vi "Model Check.vi"(8 "error in (no error)":errorcluster, 11 "VISA resource name":refnum<visa-resource-name>) -> (0 "error out":errorcluster, 1 "Model":i32(ring) items=["MSO 2000 Series", "DSO 2000 Series", "MSO 3000 Series", "DSO 3000 Series", "MSO 3000T Series", "DSO 3000T Series", "MSO 4000 Series", "DSO 4000 Series", "MSO 6000 Series", "DSO 6000 Series", "1000 Series"], 2 "Not 2000 or 3000 Series":bool, 3 "VISA resource name out":refnum<visa-resource-name>)   [LabVIEW 2023, in "Keysight-DSQx3014T.lvlib"]
doc: "Checks whether the instrument is Agilent InfiniiVision 4000 X-Series Oscilloscopes or not."
uses:
  Keysight-DSQx3014T.lvlib
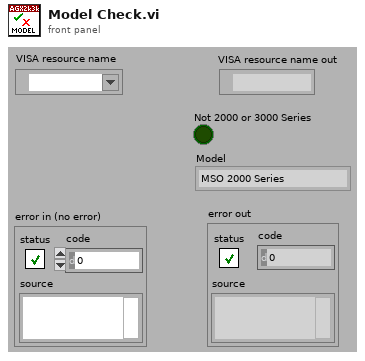
[diagram p1: front panel]
types:
  T1 = typedef "Keysight-DSQx3014T.lvlib/Extended User Data.ctl" = cluster{"X-Series Mode":u16, "Acquisition Type (0: Normal)":i32}
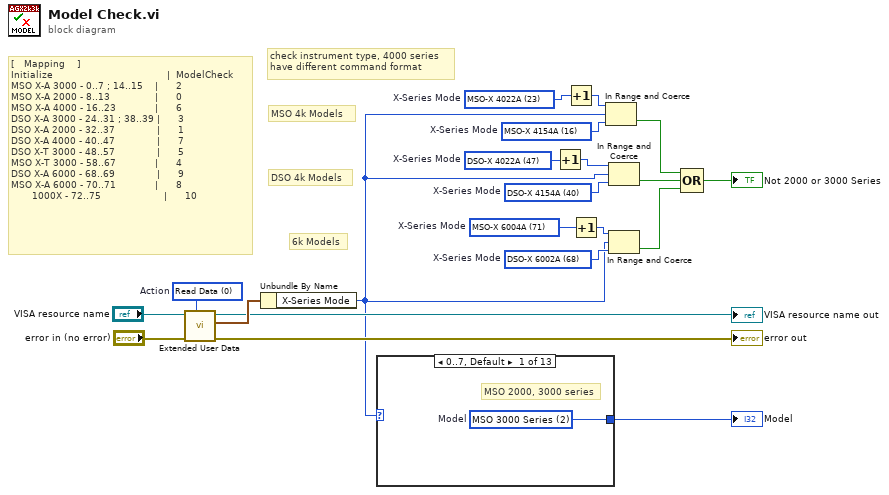
[diagram p0: block diagram]
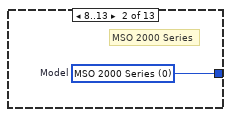
[diagram p2: hidden frame]
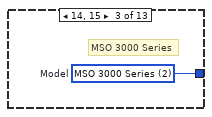
[diagram p3: hidden frame]
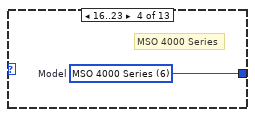
[diagram p4: hidden frame]
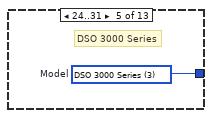
[diagram p5: hidden frame]
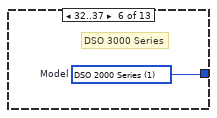
[diagram p6: hidden frame]
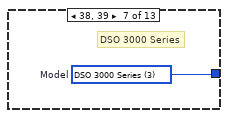
[diagram p7: hidden frame]
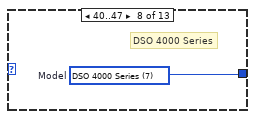
[diagram p8: hidden frame]
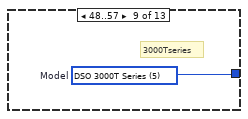
[diagram p9: hidden frame]
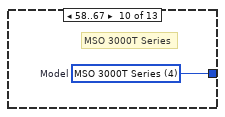
[diagram p10: hidden frame]
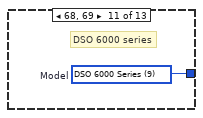
[diagram p11: hidden frame]
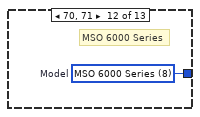
[diagram p12: hidden frame]
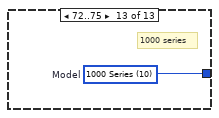
[diagram p13: hidden frame]
diagram:
  w9 = u16 68 items=["MSO-X 3014A", "MSO-X 3024A", "MSO-X 3034A", "MSO-X 3054A", "MSO-X 3012A", "MSO-X 3022A", "MSO-X 3032A", "MSO-X 3052A", "MSO-X 2004A", "MSO-X 2014A", "MSO-X 2024A", "MSO-X 2002A", "MSO-X 2012A", "MSO-X 2022A", "MSO-X 3104A", "MSO-X 3102A", "MSO-X 4154A", "MSO-X 4104A", "MSO-X 4054A", "MSO-X 4034A", "MSO-X 4024A", "MSO-X 4052A", "MSO-X 4032A", "MSO-X 4022A", "DSO-X 3014A", "DSO-X 3024A", "DSO-X 3034A", "DSO-X 3054A", "DSO-X 3012A", "DSO-X 3022A", "DSO-X 3032A", "DSO-X 3052A", "DSO-X 2004A", "DSO-X 2014A", "DSO-X 2024A", "DSO-X 2002A", "DSO-X 2012A", "DSO-X 2022A", "DSO-X 3104A", "DSO-X 3102A", "DSO-X 4154A", "DSO-X 4104A", "DSO-X 4054A", "DSO-X 4034A", "DSO-X 4024A", "DSO-X 4052A", "DSO-X 4032A", "DSO-X 4022A", "DSO-X 3012T", "DSO-X 3014T", "DSO-X 3022T", "DSO-X 3024T", "DSO-X 3032T", "DSO-X 3034T", "DSO-X 3052T", "DSO-X 3054T", "DSO-X 3102T", "DSO-X 3104T", "MSO-X 3012T", "MSO-X 3014T", "MSO-X 3022T", "MSO-X 3024T", "MSO-X 3032T", "MSO-X 3034T", "MSO-X 3052T", "MSO-X 3054T", "MSO-X 3102T", "MSO-X 3104T", "DSO-X 6002A", "DSO-X 6004A", "MSO-X 6002A", "MSO-X 6004A"]  # X-Series Mode
  w14 = u16 40 items=["MSO-X 3014A", "MSO-X 3024A", "MSO-X 3034A", "MSO-X 3054A", "MSO-X 3012A", "MSO-X 3022A", "MSO-X 3032A", "MSO-X 3052A", "MSO-X 2004A", "MSO-X 2014A", "MSO-X 2024A", "MSO-X 2002A", "MSO-X 2012A", "MSO-X 2022A", "MSO-X 3104A", "MSO-X 3102A", "MSO-X 4154A", "MSO-X 4104A", "MSO-X 4054A", "MSO-X 4034A", "MSO-X 4024A", "MSO-X 4052A", "MSO-X 4032A", "MSO-X 4022A", "DSO-X 3014A", "DSO-X 3024A", "DSO-X 3034A", "DSO-X 3054A", "DSO-X 3012A", "DSO-X 3022A", "DSO-X 3032A", "DSO-X 3052A", "DSO-X 2004A", "DSO-X 2014A", "DSO-X 2024A", "DSO-X 2002A", "DSO-X 2012A", "DSO-X 2022A", "DSO-X 3104A", "DSO-X 3102A", "DSO-X 4154A", "DSO-X 4104A", "DSO-X 4054A", "DSO-X 4034A", "DSO-X 4024A", "DSO-X 4052A", "DSO-X 4032A", "DSO-X 4022A", "DSO-X 3012T", "DSO-X 3014T", "DSO-X 3022T", "DSO-X 3024T", "DSO-X 3032T", "DSO-X 3034T", "DSO-X 3052T", "DSO-X 3054T", "DSO-X 3102T", "DSO-X 3104T", "MSO-X 3012T", "MSO-X 3014T", "MSO-X 3022T", "MSO-X 3024T", "MSO-X 3032T", "MSO-X 3034T", "MSO-X 3052T", "MSO-X 3054T", "MSO-X 3102T", "MSO-X 3104T", "DSO-X 6002A", "DSO-X 6004A", "MSO-X 6002A", "MSO-X 6004A"]  # X-Series Mode
  w15 = u16 16 items=["MSO-X 3014A", "MSO-X 3024A", "MSO-X 3034A", "MSO-X 3054A", "MSO-X 3012A", "MSO-X 3022A", "MSO-X 3032A", "MSO-X 3052A", "MSO-X 2004A", "MSO-X 2014A", "MSO-X 2024A", "MSO-X 2002A", "MSO-X 2012A", "MSO-X 2022A", "MSO-X 3104A", "MSO-X 3102A", "MSO-X 4154A", "MSO-X 4104A", "MSO-X 4054A", "MSO-X 4034A", "MSO-X 4024A", "MSO-X 4052A", "MSO-X 4032A", "MSO-X 4022A", "DSO-X 3014A", "DSO-X 3024A", "DSO-X 3034A", "DSO-X 3054A", "DSO-X 3012A", "DSO-X 3022A", "DSO-X 3032A", "DSO-X 3052A", "DSO-X 2004A", "DSO-X 2014A", "DSO-X 2024A", "DSO-X 2002A", "DSO-X 2012A", "DSO-X 2022A", "DSO-X 3104A", "DSO-X 3102A", "DSO-X 4154A", "DSO-X 4104A", "DSO-X 4054A", "DSO-X 4034A", "DSO-X 4024A", "DSO-X 4052A", "DSO-X 4032A", "DSO-X 4022A", "DSO-X 3012T", "DSO-X 3014T", "DSO-X 3022T", "DSO-X 3024T", "DSO-X 3032T", "DSO-X 3034T", "DSO-X 3052T", "DSO-X 3054T", "DSO-X 3102T", "DSO-X 3104T", "MSO-X 3012T", "MSO-X 3014T", "MSO-X 3022T", "MSO-X 3024T", "MSO-X 3032T", "MSO-X 3034T", "MSO-X 3052T", "MSO-X 3054T", "MSO-X 3102T", "MSO-X 3104T", "DSO-X 6002A", "DSO-X 6004A", "MSO-X 6002A", "MSO-X 6004A"]  # X-Series Mode
  w7 = u16 71 items=["MSO-X 3014A", "MSO-X 3024A", "MSO-X 3034A", "MSO-X 3054A", "MSO-X 3012A", "MSO-X 3022A", "MSO-X 3032A", "MSO-X 3052A", "MSO-X 2004A", "MSO-X 2014A", "MSO-X 2024A", "MSO-X 2002A", "MSO-X 2012A", "MSO-X 2022A", "MSO-X 3104A", "MSO-X 3102A", "MSO-X 4154A", "MSO-X 4104A", "MSO-X 4054A", "MSO-X 4034A", "MSO-X 4024A", "MSO-X 4052A", "MSO-X 4032A", "MSO-X 4022A", "DSO-X 3014A", "DSO-X 3024A", "DSO-X 3034A", "DSO-X 3054A", "DSO-X 3012A", "DSO-X 3022A", "DSO-X 3032A", "DSO-X 3052A", "DSO-X 2004A", "DSO-X 2014A", "DSO-X 2024A", "DSO-X 2002A", "DSO-X 2012A", "DSO-X 2022A", "DSO-X 3104A", "DSO-X 3102A", "DSO-X 4154A", "DSO-X 4104A", "DSO-X 4054A", "DSO-X 4034A", "DSO-X 4024A", "DSO-X 4052A", "DSO-X 4032A", "DSO-X 4022A", "DSO-X 3012T", "DSO-X 3014T", "DSO-X 3022T", "DSO-X 3024T", "DSO-X 3032T", "DSO-X 3034T", "DSO-X 3052T", "DSO-X 3054T", "DSO-X 3102T", "DSO-X 3104T", "MSO-X 3012T", "MSO-X 3014T", "MSO-X 3022T", "MSO-X 3024T", "MSO-X 3032T", "MSO-X 3034T", "MSO-X 3052T", "MSO-X 3054T", "MSO-X 3102T", "MSO-X 3104T", "DSO-X 6002A", "DSO-X 6004A", "MSO-X 6002A", "MSO-X 6004A"]  # X-Series Mode
  w6 = u16 23 items=["MSO-X 3014A", "MSO-X 3024A", "MSO-X 3034A", "MSO-X 3054A", "MSO-X 3012A", "MSO-X 3022A", "MSO-X 3032A", "MSO-X 3052A", "MSO-X 2004A", "MSO-X 2014A", "MSO-X 2024A", "MSO-X 2002A", "MSO-X 2012A", "MSO-X 2022A", "MSO-X 3104A", "MSO-X 3102A", "MSO-X 4154A", "MSO-X 4104A", "MSO-X 4054A", "MSO-X 4034A", "MSO-X 4024A", "MSO-X 4052A", "MSO-X 4032A", "MSO-X 4022A", "DSO-X 3014A", "DSO-X 3024A", "DSO-X 3034A", "DSO-X 3054A", "DSO-X 3012A", "DSO-X 3022A", "DSO-X 3032A", "DSO-X 3052A", "DSO-X 2004A", "DSO-X 2014A", "DSO-X 2024A", "DSO-X 2002A", "DSO-X 2012A", "DSO-X 2022A", "DSO-X 3104A", "DSO-X 3102A", "DSO-X 4154A", "DSO-X 4104A", "DSO-X 4054A", "DSO-X 4034A", "DSO-X 4024A", "DSO-X 4052A", "DSO-X 4032A", "DSO-X 4022A", "DSO-X 3012T", "DSO-X 3014T", "DSO-X 3022T", "DSO-X 3024T", "DSO-X 3032T", "DSO-X 3034T", "DSO-X 3052T", "DSO-X 3054T", "DSO-X 3102T", "DSO-X 3104T", "MSO-X 3012T", "MSO-X 3014T", "MSO-X 3022T", "MSO-X 3024T", "MSO-X 3032T", "MSO-X 3034T", "MSO-X 3052T", "MSO-X 3054T", "MSO-X 3102T", "MSO-X 3104T", "DSO-X 6002A", "DSO-X 6004A", "MSO-X 6002A", "MSO-X 6004A"]  # X-Series Mode
  w4 = u16 47 items=["MSO-X 3014A", "MSO-X 3024A", "MSO-X 3034A", "MSO-X 3054A", "MSO-X 3012A", "MSO-X 3022A", "MSO-X 3032A", "MSO-X 3052A", "MSO-X 2004A", "MSO-X 2014A", "MSO-X 2024A", "MSO-X 2002A", "MSO-X 2012A", "MSO-X 2022A", "MSO-X 3104A", "MSO-X 3102A", "MSO-X 4154A", "MSO-X 4104A", "MSO-X 4054A", "MSO-X 4034A", "MSO-X 4024A", "MSO-X 4052A", "MSO-X 4032A", "MSO-X 4022A", "DSO-X 3014A", "DSO-X 3024A", "DSO-X 3034A", "DSO-X 3054A", "DSO-X 3012A", "DSO-X 3022A", "DSO-X 3032A", "DSO-X 3052A", "DSO-X 2004A", "DSO-X 2014A", "DSO-X 2024A", "DSO-X 2002A", "DSO-X 2012A", "DSO-X 2022A", "DSO-X 3104A", "DSO-X 3102A", "DSO-X 4154A", "DSO-X 4104A", "DSO-X 4054A", "DSO-X 4034A", "DSO-X 4024A", "DSO-X 4052A", "DSO-X 4032A", "DSO-X 4022A", "DSO-X 3012T", "DSO-X 3014T", "DSO-X 3022T", "DSO-X 3024T", "DSO-X 3032T", "DSO-X 3034T", "DSO-X 3052T", "DSO-X 3054T", "DSO-X 3102T", "DSO-X 3104T", "MSO-X 3012T", "MSO-X 3014T", "MSO-X 3022T", "MSO-X 3024T", "MSO-X 3032T", "MSO-X 3034T", "MSO-X 3052T", "MSO-X 3054T", "MSO-X 3102T", "MSO-X 3104T", "DSO-X 6002A", "DSO-X 6004A", "MSO-X 6002A", "MSO-X 6004A"]  # X-Series Mode
  w21 = 0 items=["Read Data", "Write Data", "Clear Data", "Clear ALL Data"]  # Action
  # "[   Mapping\t   ]\nInitialize                                      |  ModelCheck\nMSO X-A 3000 - 0..7 ; 14..15\t   |      2\nMSO X-A 2000 - 8..13\t              |      0      \nMSO X-A 4000 - 16..23\t            |      6\nDSO X-A 3000 - 24..31 ; 38..39 |\t     3\nDSO X-A 2000 - 32..37\t             |      1\nDSO X-A 4000 - 40..47\t             |      7\nDSO X-T 3000 - 48..57\t             |      5\nMSO X-T 3000 - 58..67\t            |      4\nDSO X-A 6000 - 68..69\t             |      9\nMSO X-A 6000 - 70..71\t            |      8\n       1000X - 72..75\t                    |      10"
  # "6k Models"
  # "DSO 4k Models"
  # "MSO 4k Models"
  # "check instrument type, 4000 series \nhave different command format"
  n1 = call "Extended User Data.vi"("Action (1: Write Data)"=w21, "error in (no error)"="error in (no error)", "VISA resource name in"="VISA resource name") -> ("error out"=→"error out":errorcluster, "User Data Out"=w20:T1, "VISA resource name out"=→"VISA resource name out":refnum<visa-resource-name>)  [unwired: 1 in, 5 out]
  n2 = Unbundle By Name(w20) -> ("X-Series Mode"=w2:u16)
  n3 = case shown="0..7, Default" w2 {
    tunnel: [w22 w23 w24 w25 w26 w27 w28 w29 w30 w31 w32 w33 w34] -> w1
    frame 0..7, Default {
      w22 = 2 items=["MSO 2000 Series", "DSO 2000 Series", "MSO 3000 Series", "DSO 3000 Series", "MSO 3000T Series", "DSO 3000T Series", "MSO 4000 Series", "DSO 4000 Series", "MSO 6000 Series", "DSO 6000 Series", "1000 Series"]  # Model
      # "MSO 2000, 3000 series"
    }
    frame 8..13 {
      w23 = 0 items=["MSO 2000 Series", "DSO 2000 Series", "MSO 3000 Series", "DSO 3000 Series", "MSO 3000T Series", "DSO 3000T Series", "MSO 4000 Series", "DSO 4000 Series", "MSO 6000 Series", "DSO 6000 Series", "1000 Series"]  # Model
      # "MSO 2000 Series"
    }
    frame 14, 15 {
      w24 = 2 items=["MSO 2000 Series", "DSO 2000 Series", "MSO 3000 Series", "DSO 3000 Series", "MSO 3000T Series", "DSO 3000T Series", "MSO 4000 Series", "DSO 4000 Series", "MSO 6000 Series", "DSO 6000 Series", "1000 Series"]  # Model
      # "MSO 3000 Series"
    }
    frame 16..23 {
      w25 = 6 items=["MSO 2000", "DSO 2000", "MSO 3000", "DSO 3000", "MSO 3000T Series", "DSO 3000T Series", "MSO 4000 Series", "DSO 4000 Series", "MSO 6000 Series", "DSO 6000 Series", "1000 Series"]  # Model
      # "MSO 4000 Series"
    }
    frame 24..31 {
      w26 = 3 items=["MSO 2000 Series", "DSO 2000 Series", "MSO 3000 Series", "DSO 3000 Series", "MSO 3000T Series", "DSO 3000T Series", "MSO 4000 Series", "DSO 4000 Series", "MSO 6000 Series", "DSO 6000 Series", "1000 Series"]  # Model
      # "DSO 3000 Series"
    }
    frame 32..37 {
      w27 = 1 items=["MSO 2000 Series", "DSO 2000 Series", "MSO 3000 Series", "DSO 3000 Series", "MSO 3000T Series", "DSO 3000T Series", "MSO 4000 Series", "DSO 4000 Series", "MSO 6000 Series", "DSO 6000 Series", "1000 Series"]  # Model
      # "DSO 3000 Series"
    }
    frame 38, 39 {
      w28 = 3 items=["MSO 2000 Series", "DSO 2000 Series", "MSO 3000 Series", "DSO 3000 Series", "MSO 3000T Series", "DSO 3000T Series", "MSO 4000 Series", "DSO 4000 Series", "MSO 6000 Series", "DSO 6000 Series", "1000 Series"]  # Model
      # "DSO 3000 Series"
    }
    frame 40..47 {
      w29 = 7 items=["MSO 2000", "DSO 2000", "MSO 3000", "DSO 3000", "MSO 3000T Series", "DSO 3000T Series", "MSO 4000 Series", "DSO 4000 Series", "MSO 6000 Series", "DSO 6000 Series", "1000 Series"]  # Model
      # "DSO 4000 Series"
    }
    frame 48..57 {
      w30 = 5 items=["MSO 2000", "DSO 2000", "MSO 3000", "DSO 3000", "MSO 3000T Series", "DSO 3000T Series", "MSO 4000 Series", "DSO 4000 Series", "MSO 6000 Series", "DSO 6000 Series", "1000 Series"]  # Model
      # "3000Tseries"
    }
    frame 58..67 {
      w31 = 4 items=["MSO 2000", "DSO 2000", "MSO 3000", "DSO 3000", "MSO 3000T Series", "DSO 3000T Series", "MSO 4000 Series", "DSO 4000 Series", "MSO 6000 Series", "DSO 6000 Series", "1000 Series"]  # Model
      # "MSO 3000T Series"
    }
    frame 68, 69 {
      w32 = 9 items=["MSO 2000", "DSO 2000", "MSO 3000", "DSO 3000", "MSO 3000T Series", "DSO 3000T Series", "MSO 4000 Series", "DSO 4000 Series", "MSO 6000 Series", "DSO 6000 Series", "1000 Series"]  # Model
      # "DSO 6000 series"
    }
    frame 70, 71 {
      w33 = 8 items=["MSO 2000", "DSO 2000", "MSO 3000", "DSO 3000", "MSO 3000T Series", "DSO 3000T Series", "MSO 4000 Series", "DSO 4000 Series", "MSO 6000 Series", "DSO 6000 Series", "1000 Series"]  # Model
      # "MSO 6000 Series"
    }
    frame 72..75 {
      w34 = 10 items=["MSO 2000 Series", "DSO 2000 Series", "MSO 3000 Series", "DSO 3000 Series", "MSO 3000T Series", "DSO 3000T Series", "MSO 4000 Series", "DSO 4000 Series", "MSO 6000 Series", "DSO 6000 Series", "1000 Series"]  # Model
      # "1000 series"
    }
  }
  "Model" <- w1
  n4 = Increment(x=w4) -> (x+1=w3:u16)
  n5 = Increment(x=w6) -> (x+1=w5:u16)
  n6 = Increment(x=w7) -> (x+1=w8:u16)
  n7 = In Range and Coerce(upper limit=w5, x=w2, lower limit=w15) -> (In Range?=w13:bool)  [unwired: 1 out]
  n8 = In Range and Coerce(upper limit=w3, x=w2, lower limit=w14) -> (In Range?=w12:bool)  [unwired: 1 out]
  n9 = In Range and Coerce(upper limit=w8, x=w2, lower limit=w9) -> (In Range?=w11:bool)  [unwired: 1 out]
  n10 = Compound Arithmetic op=OR(w13, w12, w11) -> (→"Not 2000 or 3000 Series":bool)
